vi "SOUR_POW_CORR_COLL_AVER_COUN.vi"(0 "VISA IN":refnum<visa-resource-name>, 5 "error in":errorcluster, 7 "Max number of readings":i32) -> (14 "VISA Out":refnum<visa-resource-name>, 19 "error out":errorcluster)   [LabVIEW 2018, in "PNA-X.lvlib"]
doc: "SOURce:POWer:CORRection:COLLect:AVERage[:COUNt] <num> \n1836\n\n(Read-Write) This command, along with SOUR:POW:CORR:COLL:AVER:NTOLerance, allows for \nsettling of the power sensor READINGS. \nSpecifies the maximum number of power readings that are taken at each stimulus point to allow for \nmeasurement settling. Each reading is averaged with the previous readings at that stimulus point. \nWhen this average meets the Average:NTOLerance value or this number of readings has been made, \nthe average is returned as the valid reading. \nThis setting is not necessary when using a PNA receiver (SOUR:POW:CORR:COLL REC) to make \nthe measurement. \nLearn more. \nParameters \n<num> Maximum number of readings to make to allow for settling. Choose any \nnumber between 3 and 25. \nExamples SOUR:POW:CORR:COLL:AVER 2 \nsource:power:correction:collect:average:count 3 \nQuery Syntax SOURce:POWer:CORRection:COLLect:AVERage[:COUNt]? \nReturn Type Numeric \nDefault 3"
uses:
  PNA-X.lvlib
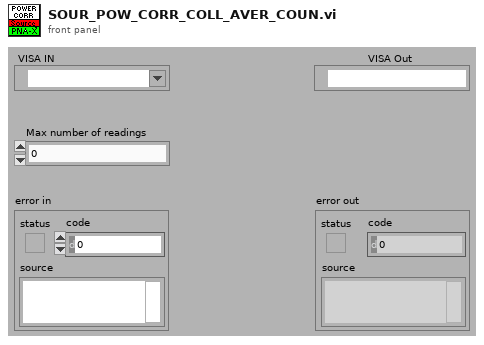
[diagram p1: front panel]
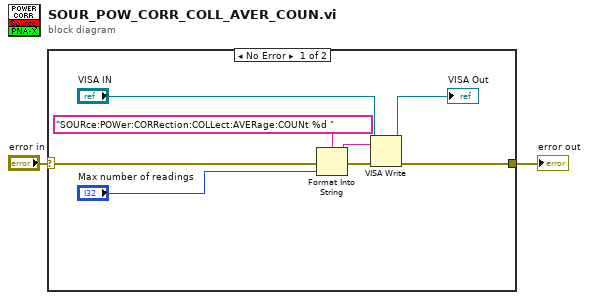
[diagram p0: block diagram]
diagram:
  n1 = case shown="No Error" "error in" {
    selector: "error in" -> [w10 w11]
    tunnel: [w5 w11] -> w1
    frame No Error {
      n2 = Format Into String(format string="SOURce:POWer:CORRection:COLLect:AVERage:COUNt %d " ("Cmdline"), error in=w10, "Max number of readings") -> (resulting string=w8:string, error out=w9:errorcluster)  [unwired: 1 in]
      n3 = VISA Write(VISA resource name="VISA IN", write buffer=w8, error in (no error)=w9) -> (VISA resource name out=→"VISA Out":refnum<visa-resource-name>, error out=w5:errorcluster)  [unwired: 1 out]
    }
    frame Error {
    }
  }
  "error out" <- w1
